vi "B2G1_host_db_logging.vi"() -> ()   [LabVIEW 2011]
uses:
  B2G1_host_db_log_vars.ctl
  <vilib>/addons/database/Connection.llb/Conn ObjectReference.ctl
  Output - Cluster b2g1.ctl
  <vilib>/Platform/TimedLoop/XDataNode/timing_clust.ctl
  <vilib>/Platform/TimedLoop/XDataNode/nitl_modes.ctl
  <vilib>/Platform/TimedLoop/XDataNode/wakeup.ctl
  <vilib>/Platform/TimedLoop/XDataNode/XDataNode.xnode
  <vilib>/Platform/TimedLoop/XDataNode/XDNodeRunTimeDep.lvlib
  <vilib>/addons/database/NI_Database_API.lvlib
  <userlib>/_JGCODE/error_logger/_error_logger.llb/ErrorLogger.lvclass
panel:
  out "target connection":bool
  out "db connection":bool
  in  "stop":bool caption="EXIT"
  in  "prefix for tables":string(combo)="B2G1"
  in  "interval [s]":u32=10 min=1 step=1
  in  "path":path
  # "B2G 1 DB Logging"
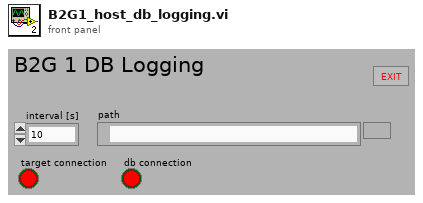
[diagram p1: front panel]
types:
  T1 = typedef "Output - Cluster b2g1.ctl" = cluster{"DFS-1 [dl]":u64, "FS-3 [l]":dbl, "DFS-1 [l/min]":dbl, "DS-1 [bar]":dbl, "V-10 ZU":bool, "V-14 ZU":bool, "FS-1 [l]":dbl, "FS-2 [l]":dbl, "TS-4 [°C]":dbl, "HS-1":bool, "V-13 [%]":u8, "V-15 [%]":u8, "P-4 [%]":u8, "P-5 [%]":u8, "Dosierung":bool, "MR Max Füllstand":bool, "MR Min Füllstand":bool, "Dosiermenge [l]":sgl, "V-14 AUF":bool, "V-10 AUF":bool, "T-1 Max Füllstand":bool, "T-1 Min Füllstand":bool, "T-2 Max Füllstand":bool, "T-2 Min Füllstand":bool, "pHS-1 [pH]":dbl, "P-4 RUN":bool, "P-5 RUN ":bool, "V-33 AUF":bool, "V-33 ZU":bool, "V-34 AUF":bool, "V-34 ZU":bool, "P-4 ERR":bool, "P-5 ERR":bool, "TS-5 [°C]":dbl, "TS-6 [°C]":dbl, "P-9 RUN":bool, "HS-2":bool}
  T2 = typedef "B2G1_host_db_log_vars.ctl" = cluster{"db timing":i64, "DFS-1":u64, "db reference":T3, "P4 RUN":bool, "P5 RUN":bool, "db logging":bool, "data refnum":refnum<k21>, "input refnum":refnum<k21>, "feeding":bool, "feeding start volume":u64, "feeding start time":timestamp, "flashing":bool, "flashing start volume":u64, "flashing start time":timestamp, "V-33":bool, "V-34":bool, "V-15":u8, "V-13":u8, "P4 ERR":bool, "P5 ERR":bool, "V-14":bool, "V-10":bool, "prefix":string, "output cluster reading time":timestamp, "HS1":bool, "P9 RUN":bool, "db connection":bool}
  T3 = typedef "NI_Database_API.lvlib/Conn ObjectReference.ctl" = refnum<k1>
  T4 = typedef "XDNodeRunTimeDep.lvlib/timing_clust.ctl" = cluster{"Expected End [f-1]":u64, "Actual End [f-1]":u64, "Finished Late? [f-1]":bool, "Expected End [i-1]":u64, "Actual End [i-1]":u64, "Finished Late? [i-1]":bool, "Expected Start [i]":u64, "Actual Start [i]":u64, "Expected Start [f]":u64, "Actual Start [f]":u64, "Source Name":string, "Structure Name":string, "Period":i64, "Deadline":i64, "Offset":i64, "Start":i64, "Priority":i32, "Timeout":i32, "Mode":T5, "Wakeup Reason":T6, "Error":errorcluster, "Source Type":string, "Secondary Source Type":string, "Global End Time":u64, "Global Start Time":u64, "Frame Duration":u64, "Iteration Duration":u64, "Assigned CPU":i32, "I/O Scan Engine Mode":u32}
  T5 = typedef "XDNodeRunTimeDep.lvlib/nitl_modes.ctl" = enum32{"No Change", "Process missed periods, maintain original phase", "Discard missed periods, maintain original phase", "Process missed periods, ignore original phase", "Discard missed periods, ignore original phase"}
  T6 = typedef "XDNodeRunTimeDep.lvlib/wakeup.ctl" = enum32{"Normal", "Aborted", "Asynchronous wakeup", "Timing source error", "Timed loop error", "Timeout"}
  T7 = enum32{"invalid app kind", "Development System", "Run Time System", "Student Edition", "Embedded LabVIEW", "Evaluation", "Custom"}
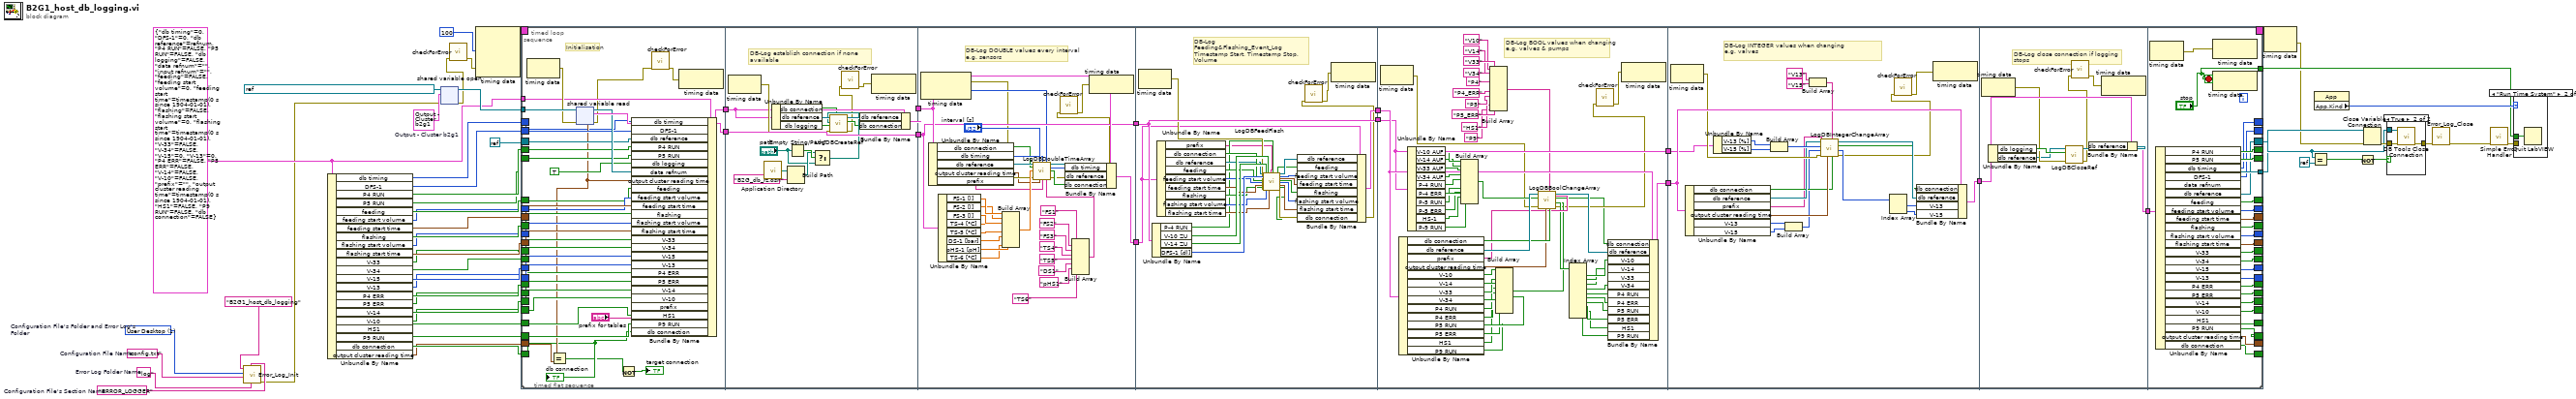
[diagram p0: block diagram]
diagram:
  w7 = "ERROR_LOGGER"  # Configuration File's Section Name
  w8 = "config.txt"  # Configuration File Name
  w9 = "log"  # Error Log Folder Name
  w10 = 1 items=["User Home", "User Desktop", "User Documents", "User Application Data", "User Preferences", "User Temporary", "Public Documents", "Public Application Data", "Public Preferences", "System Core Libraries", "System Installed Libraries", "Application Files", "Boot Volume Root"]  # Configuration File's Folder and Error Log's Folder
  w45 = T1 {"DFS-1 [dl]"=0, "FS-3 [l]"=0.0, "DFS-1 [l/min]"=0.0, "DS-1 [bar]"=0.0, "V-10 ZU"=FALSE, "V-14 ZU"=FALSE, "FS-1 [l]"=0.0, "FS-2 [l]"=0.0, "TS-4 [°C]"=0.0, "HS-1"=FALSE, "V-13 [%]"=0, "V-15 [%]"=0, "P-4 [%]"=0, "P-5 [%]"=0, "Dosierung"=FALSE, "MR Max Füllstand"=FALSE, "MR Min Füllstand"=FALSE, "Dosiermenge [l]"=0.0, "V-14 AUF"=FALSE, "V-10 AUF"=FALSE, "T-1 Max Füllstand"=FALSE, "T-1 Min Füllstand"=FALSE, "T-2 Max Füllstand"=FALSE, "T-2 Min Füllstand"=FALSE, "pHS-1 [pH]"=0.0, "P-4 RUN"=FALSE, "P-5 RUN "=FALSE, "V-33 AUF"=FALSE, "V-33 ZU"=FALSE, "V-34 AUF"=FALSE, "V-34 ZU"=FALSE, "P-4 ERR"=FALSE, "P-5 ERR"=FALSE, "TS-5 [°C]"=0.0, "TS-6 [°C]"=0.0, "P-9 RUN"=FALSE, "HS-2"=FALSE}  # Output - Cluster b2g1
  w34 = T2 {"db timing"=0, "DFS-1"=0, "db reference"=refnum, "P4 RUN"=FALSE, "P5 RUN"=FALSE, "db logging"=FALSE, "data refnum"="", "input refnum"="", "feeding"=FALSE, "feeding start volume"=0, "feeding start time"=timestamp(0 s since 1904-01-01), "flashing"=FALSE, "flashing start volume"=0, "flashing start time"=timestamp(0 s since 1904-01-01), "V-33"=FALSE, "V-34"=FALSE, "V-15"=0, "V-13"=0, "P4 ERR"=FALSE, "P5 ERR"=FALSE, "V-14"=FALSE, "V-10"=FALSE, "prefix"="", "output cluster reading time"=timestamp(0 s since 1904-01-01), "HS1"=FALSE, "P9 RUN"=FALSE, "db connection"=FALSE} ("log vars")
  n1 = call "Error_Log_Init.vi"("Error Log Folder Name"=w9, "Configuration File's Section Name"=w7, "Configuration File Name"=w8, "Configuration File's Folder and Error Log's Folder"=w10, "Application Name (Application)"="B2G1_host_db_logging") -> ("error out"=w5:errorcluster)  [unwired: 6 in]
  n2 = Unbundle By Name(w34) -> ("db timing"=w32:i64, "DFS-1"=w33:u64, "P4 RUN"=w31:bool, "P5 RUN"=w30:bool, "feeding"=w29:bool, "feeding start volume"=w28:u64, "feeding start time"=w27:timestamp, "flashing"=w26:bool, "flashing start volume"=w25:u64, "flashing start time"=w24:timestamp, "V-33"=w23:bool, "V-34"=w22:bool, "V-15"=w21:u8, "V-13"=w20:u8, "P4 ERR"=w19:bool, "P5 ERR"=w18:bool, "V-14"=w17:bool, "V-10"=w16:bool, "HS1"=w15:bool, "P9 RUN"=w14:bool, "db connection"=w13:bool, "output cluster reading time"=w1:timestamp)
  n3 = shared-variable-open(refnum<k21> "ni.var.psp://10.27.40.24/variables - b2g1/data - network - b2g1" ("output variable"), w5, w45) -> (w46:refnum<k21>, w12:errorcluster)  [unwired: 1 in]
  n4 = call <userlib>:"checkForError.vi"("Error In"=w12) -> ("error out"=w11:errorcluster)  [unwired: 9 in, 1 out]
  n5 = node-c288(i64 100 ("Period"), w11) -> (w50:T4)  [unwired: 2 in]
  n6 = timed-loop {
    timing: w50 -> [_]
    timing-out: [_] -> w49
    shift-right: [w99] -> _
    shift-left: w32 -> [w100]
    tunnel: w34 -> [w98]
    shift-right: [w62] -> _
    shift-left: w33 -> [w90]
    shift-right: [w61] -> w38
    shift-left: refnum<k0> refnum -> [w97]
    shift-right: [w96] -> _
    shift-left: w31 -> [w95]
    shift-right: [w94] -> _
    shift-left: w30 -> [w93]
    tunnel: w46 -> [w92]
    tunnel: [w91] -> w37
    shift-right: [w89] -> _
    shift-left: w29 -> [w88]
    shift-right: [w87] -> _
    shift-left: w26 -> [w86]
    shift-right: [w85] -> _
    shift-left: w28 -> [w84]
    shift-right: [w83] -> _
    shift-left: w25 -> [w82]
    shift-right: [w81] -> _
    shift-left: w24 -> [w80]
    shift-right: [w79] -> _
    shift-left: w27 -> [w78]
    shift-right: [w77] -> _
    shift-left: w21 -> [w72]
    shift-right: [w76] -> _
    shift-left: w20 -> [w71]
    shift-right: [w75] -> _
    shift-left: w22 -> [w73]
    shift-right: [w74] -> _
    shift-left: w23 -> [w53]
    shift-right: [w70] -> _
    shift-left: w19 -> [w69]
    shift-right: [w68] -> _
    shift-left: w18 -> [w67]
    shift-right: [w66] -> _
    shift-left: w17 -> [w63]
    shift-right: [w65] -> _
    shift-left: w16 -> [w64]
    tunnel: [w60] -> w36
    shift-right: [w59] -> _
    shift-left: w15 -> [w58]
    shift-right: [w57] -> _
    shift-left: w14 -> [w56]
    shift-right: [w55] -> _
    shift-left: w1 -> [w54]
    shift-right: [w52] -> _
    shift-left: w13 -> [w51]
    stop <- "stop" stop-if-true
    n7 = timed-sequence {
      timing: _ -> [_]
      timing-out: _ -> [_]
      tunnel: w100 -> [w162]
      tunnel: [w161] -> w99
      tunnel: w98 -> [w160]
      tunnel: w97 -> [w159]
      tunnel: [w158] -> w96
      tunnel: w95 -> [w157]
      tunnel: [w156] -> w94
      tunnel: w93 -> [w155]
      tunnel: w92 -> [w150]
      tunnel: [w149] -> w91
      tunnel: w90 -> [w148]
      tunnel: [w145] -> w89
      tunnel: w88 -> [w144]
      tunnel: [w143] -> w87
      tunnel: w86 -> [w142]
      tunnel: [w141] -> w85
      tunnel: w84 -> [w140]
      tunnel: [w139] -> w83
      tunnel: w82 -> [w138]
      tunnel: [w137] -> w81
      tunnel: w80 -> [w136]
      tunnel: [w135] -> w79
      tunnel: w78 -> [w134]
      tunnel: [w131] -> w77
      tunnel: [w130] -> w76
      tunnel: [w129] -> w75
      tunnel: [w128] -> w74
      tunnel: w73 -> [w127]
      tunnel: w72 -> [w126]
      tunnel: w71 -> [w125]
      tunnel: [w122] -> w70
      tunnel: w69 -> [w121]
      tunnel: [w120] -> w68
      tunnel: w67 -> [w119]
      tunnel: [w118] -> w66
      tunnel: [w117] -> w65
      tunnel: w64 -> [w116]
      tunnel: w63 -> [w115]
      tunnel: [w112] -> w62
      tunnel: [w111] -> w61
      tunnel: [w110] -> w60
      tunnel: [w109] -> w59
      tunnel: w58 -> [w108]
      tunnel: [w107] -> w57
      tunnel: w56 -> [w106]
      tunnel: [w105] -> w55
      tunnel: w54 -> [w104]
      tunnel: w53 -> [w103]
      tunnel: [w102] -> w52
      tunnel: w51 -> [w101]
      n8 = timed-flat-sequence {
        tunnel: w162 -> [w168]
        tunnel: [w196] -> w154
        tunnel: w160 -> [w180]
        tunnel: [w179] -> w152
        tunnel: w159 -> [w182]
        tunnel: w157 -> [w183]
        tunnel: w155 -> [w184]
        tunnel: w150 -> [w198]
        tunnel: w148 -> [w181]
        tunnel: w144 -> [w186]
        tunnel: w142 -> [w189]
        tunnel: w140 -> [w187]
        tunnel: w138 -> [w190]
        tunnel: w136 -> [w191]
        tunnel: w134 -> [w188]
        tunnel: w127 -> [w193]
        tunnel: w126 -> [w194]
        tunnel: w125 -> [w195]
        tunnel: w121 -> [w178]
        tunnel: w119 -> [w177]
        tunnel: w116 -> [w175]
        tunnel: w115 -> [w176]
        tunnel: w108 -> [w173]
        tunnel: w106 -> [w172]
        tunnel: w104 -> [w170]
        tunnel: w103 -> [w192]
        tunnel: w101 -> [w166]
        tunnel: w154 -> [w220]
        tunnel: [w220] -> w153
        tunnel: w152 -> [w217]
        tunnel: [w216] -> w151
        tunnel: w153 -> [w257]
        tunnel: [w257] -> w147
        tunnel: w151 -> [w258]
        tunnel: [w259] -> w146
        tunnel: w147 -> [w292]
        tunnel: [w292] -> w133
        tunnel: w146 -> [w281]
        tunnel: [w287] -> w132
        tunnel: w133 -> [w351]
        tunnel: w132 -> [w352]
        tunnel: [w353] -> w124
        tunnel: [w351] -> w113
        tunnel: w124 -> [w381]
        tunnel: [w382] -> w123
        tunnel: w113 -> [w363]
        tunnel: w123 -> [w394]
        tunnel: [w390] -> w114
        tunnel: [w408] -> w161
        tunnel: [w426] -> w158
        tunnel: [w425] -> w156
        tunnel: [w424] -> w149
        tunnel: [w423] -> w145
        tunnel: [w420] -> w143
        tunnel: [w422] -> w141
        tunnel: [w419] -> w139
        tunnel: [w418] -> w137
        tunnel: [w421] -> w135
        tunnel: [w415] -> w131
        tunnel: [w414] -> w130
        tunnel: [w416] -> w129
        tunnel: [w417] -> w128
        tunnel: [w413] -> w122
        tunnel: [w412] -> w120
        tunnel: [w411] -> w118
        tunnel: [w410] -> w117
        tunnel: w114 -> [w409]
        tunnel: [w407] -> w112
        tunnel: [w406] -> w111
        tunnel: ["stop"] -> w110
        tunnel: [w404] -> w109
        tunnel: [w403] -> w107
        tunnel: [w402] -> w105
        tunnel: [w401] -> w102
        frame #0 {
          # "Initialisation"
          n9 = node-c288() -> (w197:errorcluster)  [unwired: 1 in]
          n10 = shared-variable-read(w198, w197) -> (w185:refnum<k21>, w164:errorcluster, w196:T1, w169:timestamp)
          n11 = Equal?(x=w169, y=w170) -> (x = y?=w165:bool)
          n12 = Not(x=w165) -> (.not. x?=→"target connection":bool)
          n13 = Bundle By Name(cluster=w180, "db timing"=w168, "DFS-1"=w181, "db reference"=w182, "P4 RUN"=w183, "P5 RUN"=w184, "db logging"=TRUE ("on/off"), "data refnum"=w185, "output cluster reading time"=w169, "feeding"=w186, "feeding start volume"=w187, "feeding start time"=w188, "flashing"=w189, "flashing start volume"=w190, "flashing start time"=w191, "V-33"=w192, "V-34"=w193, "V-15"=w194, "V-13"=w195, "P4 ERR"=w178, "P5 ERR"=w177, "V-14"=w176, "V-10"=w175, "prefix"="prefix for tables", "HS1"=w173, "P9 RUN"=w172, "db connection"=w166) -> (w179:T2)
          n14 = call <userlib>:"checkForError.vi"("Error In"=w164) -> ("error out"=w163:errorcluster)  [unwired: 9 in, 1 out]
          n15 = node-c288(w163) -> ()  [unwired: 1 out]
          "db connection" <- w166
        }
        frame #1 {
          # "DB-Log establish connection if none available"
          n16 = node-c288() -> (w218:errorcluster)  [unwired: 1 in]
          n17 = call <vilib>:"Application Directory.vi"() -> ("Application Directory"=w211:path)
          n18 = Unbundle By Name(w217) -> ("db connection"=w207:bool, "db reference"=w219:T3, "db logging"=w214:bool)
          n19 = Build Path(base path=w211, name or relative path="B2G_db_rz.dsn" ("Name of ini file 2")) -> (appended path=w212:path)
          n20 = Empty String/Path?(string/path="path") -> (empty?=w213:bool)
          n21 = Select(t=w212, s=w213, f="path") -> (s? t:f=w209:path)
          n22 = call "LogDBCreateRef.vi"("db connection"=w207, "error in (no error)"=w218, "db"=w214, "Pfad in"=w209, "Refnum in"=w219) -> ("error out"=w205:errorcluster, "db connection"=w206:bool, "Refnum out"=w215:T3)  [unwired: 4 in]
          n23 = call <userlib>:"checkForError.vi"("Error In"=w205) -> ("error out"=w204:errorcluster)  [unwired: 9 in, 1 out]
          n24 = Bundle By Name(cluster=w217, "db reference"=w215, "db connection"=w206) -> (w216:T2)
          n25 = node-c288(w204) -> ()  [unwired: 1 out]
        }
        frame #2 {
          # "DB-Log DOUBLE values every interval\ne.g. sensors"
          n26 = node-c288() -> (w233:errorcluster, w254:i64)  [unwired: 1 in]
          n27 = Unbundle By Name(w258) -> ("db connection"=w250:bool, "db timing"=w255:i64, "db reference"=w251:T3, "output cluster reading time"=w232:timestamp, "prefix"=w231:string)
          n28 = Unbundle By Name(w257) -> ("FS-1 [l]"=w241:dbl, "FS-2 [l]"=w240:dbl, "FS-3 [l]"=w239:dbl, "TS-4 [°C]"=w238:dbl, "TS-5 [°C]"=w237:dbl, "DS-1 [bar]"=w236:dbl, "pHS-1 [pH]"=w235:dbl, "TS-6 [°C]"=w229:dbl)
          n29 = Build Array(w241, w240, w239, w238, w237, w236, w235, w229) -> (w234:dbl[])
          n30 = Build Array("FS1" ("table"), "FS2" ("table"), "FS3" ("table"), "TS4" ("table"), "TS5" ("table"), "DS1" ("table"), "pHS1" ("table"), "TS6" ("table")) -> (w242:string[])
          n31 = call "LogDBDoubleTimeArray.vi"("Refnum in"=w251, "db Interval [s]"="interval [s]", "db timing"=w255, "Actual Start [f] in"=w254, "db connection"=w250, "values"=w234, "error in (no error)"=w233, "Time Stamp"=w232, "prefix"=w231, "names"=w242) -> ("Refnum out"=w252:T3, "Actual Start [f] out"=w253:i64, "db connection"=w228:bool, "error out"=w227:errorcluster)  [unwired: 2 in]
          n32 = call <userlib>:"checkForError.vi"("Error In"=w227) -> ("error out"=w226:errorcluster)  [unwired: 9 in, 1 out]
          n33 = Bundle By Name(cluster=w258, "db timing"=w253, "db reference"=w252, "db connection"=w228) -> (w259:T2)
          n34 = node-c288(w226) -> ()  [unwired: 1 out]
        }
        frame #3 {
          # "DB-Log\nFeeding&Flashing_Event_Log\nTimestamp Start, Timestamp Stop, Volume"
          n35 = node-c288() -> (w288:errorcluster)  [unwired: 1 in]
          n36 = Unbundle By Name(w292) -> ("P-4 RUN"=w270:bool, "V-10 ZU"=w290:bool, "V-14 ZU"=w289:bool, "DFS-1 [dl]"=w291:u64)
          n37 = Unbundle By Name(w281) -> ("prefix"=w269:string, "db connection"=w284:bool, "db reference"=w283:T3, "feeding"=w271:bool, "feeding start volume"=w282:u64, "feeding start time"=w280:timestamp, "flashing"=w272:bool, "flashing start volume"=w274:u64, "flashing start time"=w273:timestamp)
          n38 = call "LogDBFeedFlash.vi"("Refnum in"=w283, "value volume [dl]"=w291, "db connection"=w284, "feeding"=w271, "feeding start volume"=w282, "feeding start time"=w280, "flashing"=w272, "error in"=w288, "valve t-2 close"=w289, "flashing start volume"=w274, "valve t-1 close"=w290, "flashing start time"=w273, "prefix"=w269, "Pump"=w270) -> ("feeding"=w285:bool, "Refnum out"=w286:T3, "feeding start volume"=w278:u64, "feeding start time"=w279:timestamp, "flashing"=w276:bool, "flashing start volume"=w275:u64, "flashing start time"=w277:timestamp, "db connection"=w266:bool, "error out"=w268:errorcluster)  [unwired: 5 in]
          n39 = Bundle By Name(cluster=w281, "db reference"=w286, "feeding"=w285, "feeding start volume"=w278, "feeding start time"=w279, "flashing"=w276, "flashing start volume"=w275, "flashing start time"=w277, "db connection"=w266) -> (w287:T2)
          n40 = call <userlib>:"checkForError.vi"("Error In"=w268) -> ("error out"=w267:errorcluster)  [unwired: 9 in, 1 out]
          n41 = node-c288(w267) -> ()  [unwired: 1 out]
        }
        frame #4 {
          # "DB-Log BOOL values when changing\ne.g. valves & pumps"
          n42 = node-c288() -> (w309:errorcluster)  [unwired: 1 in]
          n43 = Unbundle By Name(w352) -> ("db connection"=w340:bool, "db reference"=w341:T3, "prefix"=w338:string, "output cluster reading time"=w339:timestamp, "V-10"=w327:bool, "V-14"=w326:bool, "V-33"=w325:bool, "V-34"=w324:bool, "P4 RUN"=w323:bool, "P4 ERR"=w322:bool, "P5 RUN"=w321:bool, "P5 ERR"=w320:bool, "HS1"=w308:bool, "P9 RUN"=w302:bool)
          n44 = Unbundle By Name(w351) -> ("V-10 AUF"=w318:bool, "V-14 AUF"=w317:bool, "V-33 AUF"=w316:bool, "V-34 AUF"=w315:bool, "P-4 RUN"=w314:bool, "P-4 ERR"=w313:bool, "P-5 RUN"=w312:bool, "P-5 ERR"=w311:bool, "HS-1"=w306:bool, "P-9 RUN"=w303:bool)
          n45 = Build Array(w318, w317, w316, w315, w314, w313, w312, w311, w306, w303) -> (w310:bool[])
          n46 = Build Array("V10" ("table"), "V14" ("table"), "V33" ("table"), "V34" ("table"), "P4" ("table"), "P4_ERR" ("table"), "P5" ("table"), "P5_ERR" ("table"), "HS1" ("table"), "P9" ("table")) -> (w342:string[])
          n47 = Build Array(w327, w326, w325, w324, w323, w322, w321, w320, w308, w302) -> (w319:bool[])
          n48 = call "LogDBBoolChangeArray.vi"("db connection"=w340, "names"=w342, "cluster reading time"=w339, "prefix"=w338, "error in (no error)"=w309, "shift reg in"=w319, "values"=w310, "db reference"=w341) -> ("error out"=w300:errorcluster, "shift reg out"=w336:bool[], "db connection"=w298:bool, "db reference out"=w337:T3)
          n49 = Index Array(array=w336) -> (element #1=w335:bool, element #2=w334:bool, element #3=w333:bool, element #4=w332:bool, element #5=w331:bool, element #6=w330:bool, element #7=w329:bool, element #8=w328:bool, element #9=w307:bool, element #10=w301:bool)  [unwired: 10 in]
          n50 = call <userlib>:"checkForError.vi"("Error In"=w300) -> ("error out"=w299:errorcluster)  [unwired: 9 in, 1 out]
          n51 = Bundle By Name(cluster=w352, "db connection"=w298, "db reference"=w337, "V-10"=w335, "V-14"=w334, "V-33"=w333, "V-34"=w332, "P4 RUN"=w331, "P4 ERR"=w330, "P5 RUN"=w329, "P5 ERR"=w328, "HS1"=w307, "P9 RUN"=w301) -> (w353:T2)
          n52 = node-c288(w299) -> ()  [unwired: 1 out]
        }
        frame #5 {
          # "DB-Log INTEGER values when changing\ne.g. valves"
          n53 = node-c288() -> (w371:errorcluster)  [unwired: 1 in]
          n54 = Unbundle By Name(w381) -> ("db connection"=w367:bool, "db reference"=w369:T3, "prefix"=w362:string, "output cluster reading time"=w370:timestamp, "V-13"=w366:u8, "V-15"=w365:u8)
          n55 = Unbundle By Name(w363) -> ("V-13 [%]"=w377:u8, "V-15 [%]"=w376:u8)
          n56 = Build Array(w377, w376) -> (w375:u8[])
          n57 = Build Array(w366, w365) -> (w364:u8[])
          n58 = Build Array("V13" ("table"), "V15" ("table")) -> (w378:string[])
          n59 = call "LogDBIntegerChangeArray.vi"("db connection"=w367, "names"=w378, "current time"=w370, "prefix"=w362, "error in (no error)"=w371, "shift reg in"=w364, "values"=w375, "Refnum in"=w369) -> ("error out"=w361:errorcluster, "shift reg out"=w372:u32[], "db connection"=w359:bool, "Refnum out"=w368:T3)
          n60 = Index Array(array=w372) -> (element #1=w374:u32, element #2=w373:u32)  [unwired: 2 in]
          n61 = call <userlib>:"checkForError.vi"("Error In"=w361) -> ("error out"=w360:errorcluster)  [unwired: 9 in, 1 out]
          n62 = Bundle By Name(cluster=w381, "db connection"=w359, "db reference"=w368, "V-13"=w374, "V-15"=w373) -> (w382:T2)
          n63 = node-c288(w360) -> ()  [unwired: 1 out]
        }
        frame #6 {
          # "DB-Log close connection if logging stops"
          n64 = node-c288() -> (w392:errorcluster)  [unwired: 1 in]
          n65 = Unbundle By Name(w394) -> ("db logging"=w393:bool, "db reference"=w391:T3)
          n66 = call "LogDBCloseRef.vi"("error in (no error)"=w392, "enable"=w393, "Refnum in"=w391) -> ("error out"=w389:errorcluster, "Refnum out"=w395:T3)  [unwired: 7 in]
          n67 = call <userlib>:"checkForError.vi"("Error In"=w389) -> ("error out"=w388:errorcluster)  [unwired: 9 in, 1 out]
          n68 = Bundle By Name(cluster=w394, "db reference"=w395) -> (w390:T2)
          n69 = node-c288(w388) -> ()  [unwired: 1 out]
        }
        frame #7 {
          n70 = node-c288() -> (w427:errorcluster)  [unwired: 1 in]
          n71 = Unbundle By Name(w409) -> ("P4 RUN"=w426:bool, "P5 RUN"=w425:bool, "db timing"=w408:i64, "DFS-1"=w407:u64, "data refnum"=w424:refnum<k21>, "db reference"=w406:T3, "feeding"=w423:bool, "feeding start volume"=w422:u64, "feeding start time"=w421:timestamp, "flashing"=w420:bool, "flashing start volume"=w419:u64, "flashing start time"=w418:timestamp, "V-33"=w417:bool, "V-34"=w416:bool, "V-15"=w415:u8, "V-13"=w414:u8, "P4 ERR"=w413:bool, "P5 ERR"=w412:bool, "V-14"=w411:bool, "V-10"=w410:bool, "HS1"=w404:bool, "P9 RUN"=w403:bool, "output cluster reading time"=w402:timestamp, "db connection"=w401:bool)
          n72 = node-c288(w427) -> ()  [unwired: 1 out]
        }
      }
    }
    n73 = node-c288() -> ()  [unwired: 1 in, 1 out]
    n74 = node-c288() -> ()  [unwired: 1 in, 1 out]
  }
  n75 = node-c288(w49) -> (w35:errorcluster)
  n76 = Equal?(x=w38, y=refnum<k0> refnum) -> (x = y?=w43:bool)
  n77 = property class="App"() -> ("App.Kind"=w39:T7)  [unwired: 2 in, 2 out]
  n78 = Not(x=w43) -> (.not. x?=w41:bool)
  n79 = Close Variable Connection(8:w35, 11:w37) -> (0:w40:errorcluster)
  n80 = case shown="True" w41 {
    tunnel: w40 -> [w435 w438]
    tunnel: w38 -> [_ w437]
    tunnel: [w435 w436] -> w4
    frame False {
    }
    frame True {
      n81 = call <vilib>:"DB Tools Close Connection.vi"("error in (no error)"=w438, "connection reference"=w437) -> ("error out"=w436:errorcluster)  [unwired: 5 in]
    }
  }
  n82 = call "Error_Log_Close.vi"("error in (no error)"=w4) -> ("error out"=w3:errorcluster)  [unwired: 10 in]
  n83 = call <vilib>:"Simple Error Handler.vi"("error in (no error)"=w3) -> ("error out"=w2:errorcluster)  [unwired: 4 in, 4 out]
  n84 = case shown="\"Run Time System\"" w39 {
    tunnel: w36 -> [_ w439 _]
    tunnel: w2 -> [_ _ _]
    frame "invalid app kind", Default {
    }
    frame "Run Time System" {
      n85 = Quit LabVIEW(quit? (T)=w439) -> ()
    }
    frame "Development System" {
    }
  }
